vi "Line Up.vi"(8 "error IO":errorcluster, 11 "Gantry In":refnum<k24>) -> (0 "error out":errorcluster, 3 "Gantry Out":refnum<k24>)   [LabVIEW 2021, in "Component Tray.lvclass"]
uses:
  Component Tray.lvclass
  C:/Program Files (x86)/Aerotech/A3200/LabVIEW/2010/Bin/Aerotech.A3200.dll
  Program Files (x86)/Aerotech/A3200/LabVIEW/2010/Bin/Aerotech.A3200.dll
  Controller/Motion/A3200/A3200.lvclass
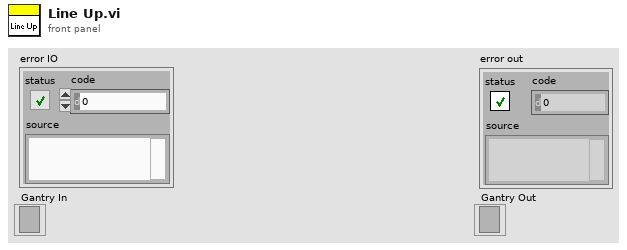
[diagram p1: front panel]
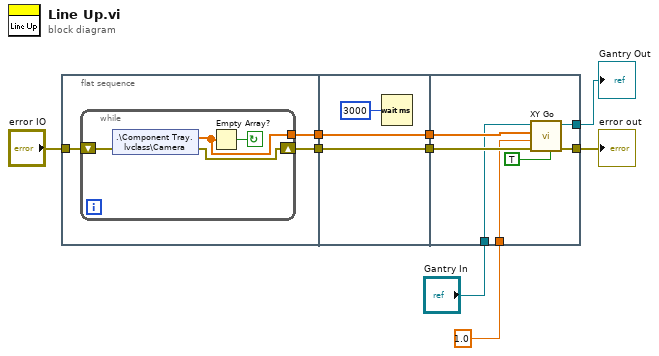
[diagram p0: block diagram]
diagram:
  n1 = flat-sequence {
    tunnel: "error IO" -> [w11]
    tunnel: [w12] -> w8
    tunnel: [w10] -> w7
    tunnel: w8 -> [w19]
    tunnel: w7 -> [w18]
    tunnel: [w19] -> w6
    tunnel: [w18] -> w5
    tunnel: w6 -> [w25]
    tunnel: w5 -> [w23]
    tunnel: 1.0 ("Speed") -> [w24]
    tunnel: "Gantry In" -> [w22]
    tunnel: [w21] -> w2
    tunnel: [w20] -> w1
    frame #0 {
      n2 = while {
        tunnel: [w14] -> w10
        shift-right: [w15] -> w12
        shift-left: w11 -> [w16]
        stop <- w13 continue-if-true
        n3 = shared-variable ".\\Component Tray.lvclass\\Camera"(error in=w16) -> (w14:dbl[], error out=w15:errorcluster)
        n4 = Empty Array?(array=w14) -> (empty?=w13:bool)
      }
    }
    frame #1 {
      n5 = Wait (ms)(milliseconds to wait=u32 3000) -> ()  [unwired: 1 out]
    }
    frame #2 {
      n6 = call "XY Go.vi"("Increment?"=TRUE, "error in (no error)"=w25, "Speed"=w24, "XY In"=w23, "Gantry In"=w22) -> ("error out"=w21:errorcluster, "Gantry Out"=w20:refnum<k24>)  [unwired: 4 in, 1 out]
    }
  }
  "error out" <- w2
  "Gantry Out" <- w1
